vi "check_has_unreacheable_square_been_formed.vi"(2 "tour_in_progress":T1[](array[typedef]), 3 "chessboard":T2[][](array[typedef])) -> (0 "unreacheable square":T1, 1 "T = unreacheable square found":bool)   [LabVIEW 2020, in "core.lvlib"]
uses:
  core.lvlib
  core_data/chess_square.ctl
  core_data/neighbour_square.ctl
  core_data/chessboard_index.ctl
  core_data/core_data.lvlib
panel:
  out "second-to-last square":T2
  # "Input\nInputs to the VI"
  # "Development\ncontrols/indicators useful for development and testing, but which are not outputs of the VI"
  # "Output\nOutputs of the VI"
  # "Description\n\nBlank VI with error handling case. \n\nSummarize the use of this VI in this space."
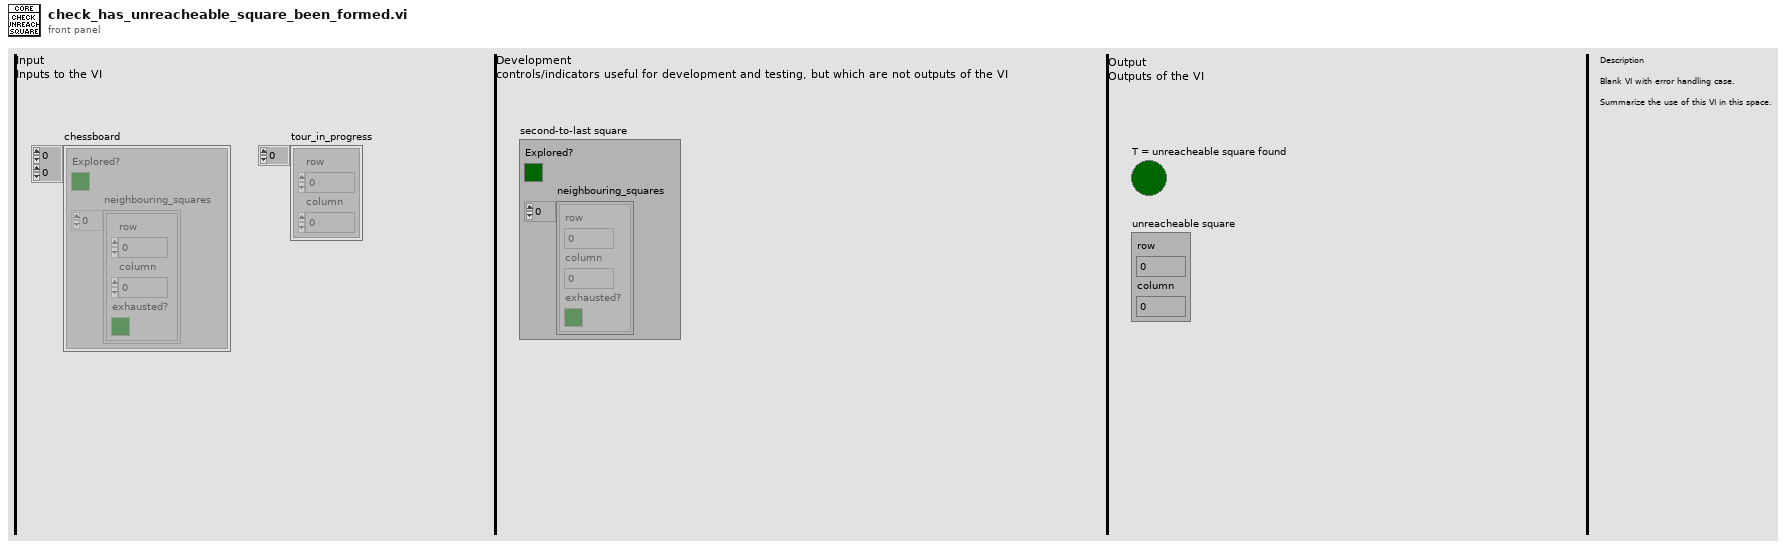
[diagram p1: front panel]
types:
  T1 = typedef "core.lvlib/core_data.lvlib/chessboard_index.ctl" = cluster{"row":u8, "column":u8}
  T2 = typedef "core.lvlib/core_data.lvlib/chess_square.ctl" = cluster{"Explored?":bool, "neighbouring_squares":T3[]}
  T3 = typedef "core.lvlib/core_data.lvlib/neighbour_square.ctl" = cluster{"row":u8, "column":u8, "exhausted?":bool}
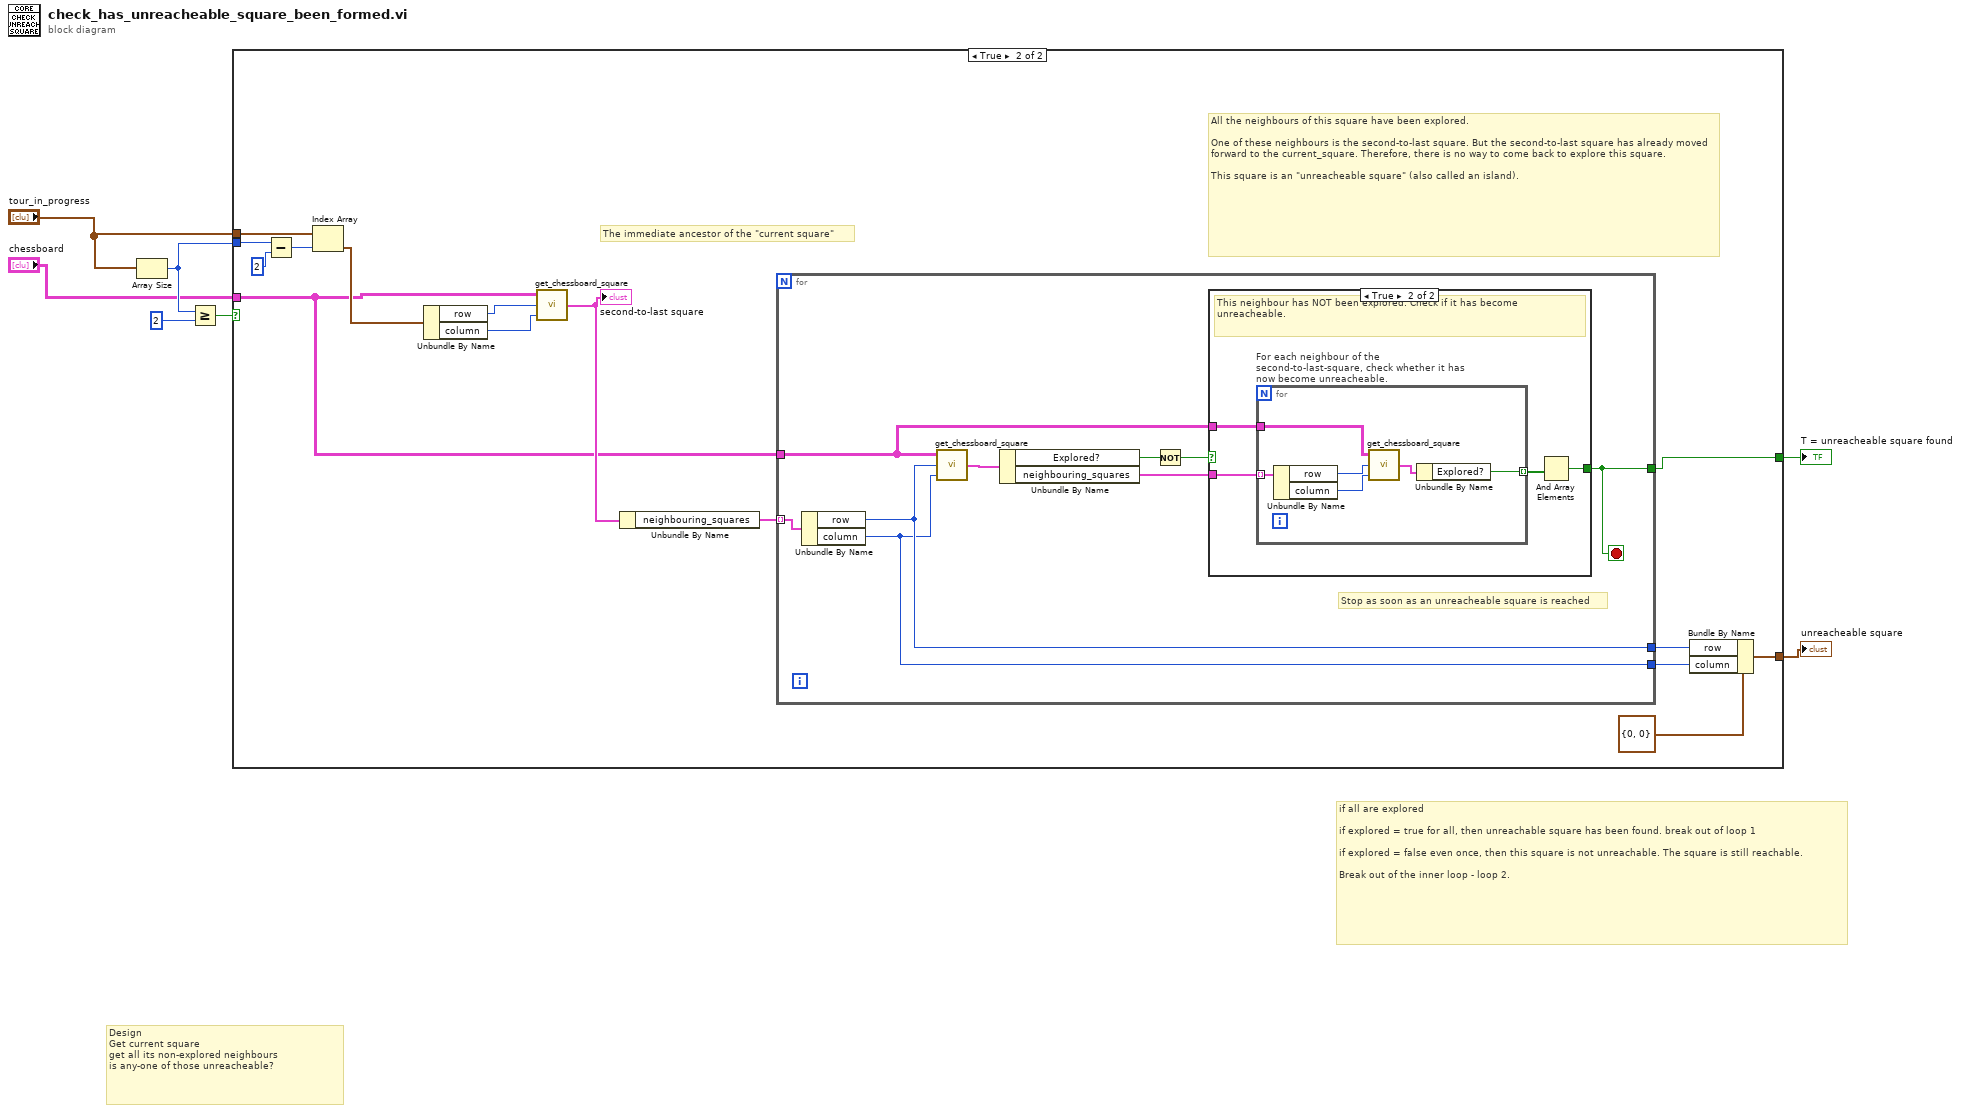
[diagram p0: block diagram]
diagram:
  # "if all are explored\n\nif explored = true for all, then unreachable square has been found. break out of loop 1\n\nif explored = false even once, then this square is not unreachable. The square is still reachable.\n\nBreak out of the inner loop - loop 2."
  # "Design\nGet current square\nget all its non-explored neighbours\nis any-one of those unreacheable?"
  n1 = Array Size(array="tour_in_progress") -> (size(s)=w7:i32)
  n2 = Greater Or Equal?(x=w7, y=2) -> (x >= y?=w4:bool)
  n3 = case shown="True" w4 {
    tunnel: "tour_in_progress" -> [_ w21]
    tunnel: "chessboard" -> [_ w15]
    tunnel: w7 -> [_ w13]
    tunnel: [_ w12] -> w5
    tunnel: [_ w8] -> w3
    frame False {
      # "This case executes when there is only one element in the \"tour_in_progress\" - the starting square."
    }
    frame True {
      # "The immediate ancestor of the \"current square\""
      # "All the neighbours of this square have been explored.\n\nOne of these neighbours is the second-to-last square. But the second-to-last square has already moved forward to the current_square. Therefore, there is no way to come back to explore this square.\n\nThis square is an \"unreacheable square\" (also called an island)."
      n4 = Subtract(x=w13, y=2 ("x")) -> (x-y=w20:i32)
      n5 = Index Array(array=w21, index=w20) -> (element=w19:T1)
      n6 = Unbundle By Name(w19) -> ("row"=w18:u8, "column"=w17:u8)
      n7 = call "get_chessboard_square.vi"("column"=w17, "row"=w18, "chessboard"=w15) -> ("chessboard_square"=w16:T2)
      "second-to-last square" <- w16
      n8 = Unbundle By Name(w16) -> ("neighbouring_squares"=w22:T3[])
      n9 = for {
        tunnel: w22 -> [w31] mode=indexing
        tunnel: w15 -> [w26]
        tunnel: [w25] -> w12
        tunnel: [w24] -> w10
        tunnel: [w23] -> w9
        stop <- w25 stop-if-true
        # "Stop as soon as an unreacheable square is reached"
        n10 = Unbundle By Name(w31) -> ("row"=w24:u8, "column"=w23:u8)
        n11 = call "get_chessboard_square.vi"("column"=w23, "row"=w24, "chessboard"=w26) -> ("chessboard_square"=w30:T2)
        n12 = Unbundle By Name(w30) -> ("Explored?"=w29:bool, "neighbouring_squares"=w27:T3[])
        n13 = Not(x=w29) -> (.not. x?=w28:bool)
        n14 = case shown="True" w28 {
          tunnel: w27 -> [_ w35]
          tunnel: w26 -> [_ w34]
          tunnel: [_ w32] -> w25
          frame False {
            # "This neighbour has been explored. It cannot be an unreacheable square."
          }
          frame True {
            # "This neighbour has NOT been explored. Check if it has become unreacheable."
            n15 = for "For each neighbour of the second-to-last-square, check whether it has now become unreacheable." {
              tunnel: w35 -> [w41] mode=indexing
              tunnel: w34 -> [w40]
              tunnel: [w36] -> w33 mode=indexing
              n16 = Unbundle By Name(w41) -> ("row"=w39:u8, "column"=w38:u8)
              n17 = call "get_chessboard_square.vi"("column"=w38, "row"=w39, "chessboard"=w40) -> ("chessboard_square"=w37:T2)
              n18 = Unbundle By Name(w37) -> ("Explored?"=w36:bool)
            }
            n19 = And Array Elements(Boolean array=w33) -> (logical AND=w32:bool)
          }
        }
      }
      n20 = Bundle By Name(cluster=T1 {"row"=0, "column"=0} ("element"), "row"=w10, "column"=w9) -> (w8:T1)
    }
  }
  "T = unreacheable square found" <- w5
  "unreacheable square" <- w3
